vi "RDS Log Reader.vi"() -> ()   [LabVIEW 2015]
uses:
  Actors/RDS Logger Actor/RDS Logger Actor/RDS Logger Actor/Logger Header.ctl
  RDS State Tracker/RDS State/RDS State.lvclass
  Libraries/RDS Child Messages/Mission Messages/Mission Controller State Control.ctl
  RDS Mission Controller Actor/Mission Controller Navigation State.ctl
  RDS Mission Controller Actor/MissionOp.ctl
  RDS State Tracker/RDS State/RDS State.lvclass/RDS State.ctl
  <vilib>/Waveform/WDTFileIO.llb/Export Waveforms To Spreadsheet File (1D).vi
  Log/Log Waveform Processors.lvlib
  RDS Mission Controller Actor/RDS Mission Controller Actor.lvlib
  Libraries/RDS Child Messages/Mission Messages/Mission Controller State Message.lvclass
panel:
  out "Open Log Path":path caption="selected path"
  out "log folder":path caption="selected path"
  in  "Browse Files":bool
  in  "Tree":string(tree)
  in  "Open":bool
  in  "Tab Control":T1(tab)
  out "Battery WF":waveform(dbl)[](graph)
  in  "Batt_Autoscale Y":bool caption="OK Button"
  in  "Nav_Autoscale Y":bool caption="OK Button"
  out "Nav WF":waveform(dbl)[](graph)
  out "Helm":waveform(dbl)[](graph)
  in  "Helm Autoscale Y":bool caption="OK Button"
  out "Speed":waveform(dbl)(graph)
  in  "STBD MCB Autoscale Y":bool caption="OK Button"
  out "STBD WFs":waveform(dbl)[](graph)
  out "Port WFs":waveform(dbl)[](graph)
  in  "Port MCB Autoscale Y":bool caption="OK Button"
  out "Thermal WFs":waveform(dbl)[](graph)
  in  "Thermal Autoscale":bool caption="OK Button"
  out "XY Graph":T2(graph)
  in  "Numeric":i32
  in  "btn_index_mission":bool caption="OK Button"
  out "Mission Controller State":T3 {"Mission"."GPS Longitude" format="%.6g"; "Mission"."GPS Latitude" format="%.6g"}
  out "Mission":refnum<class "RDS State.lvclass">[](array[class])
  out "Header":T6
  in  "stop":bool
  out "size(s)":i32
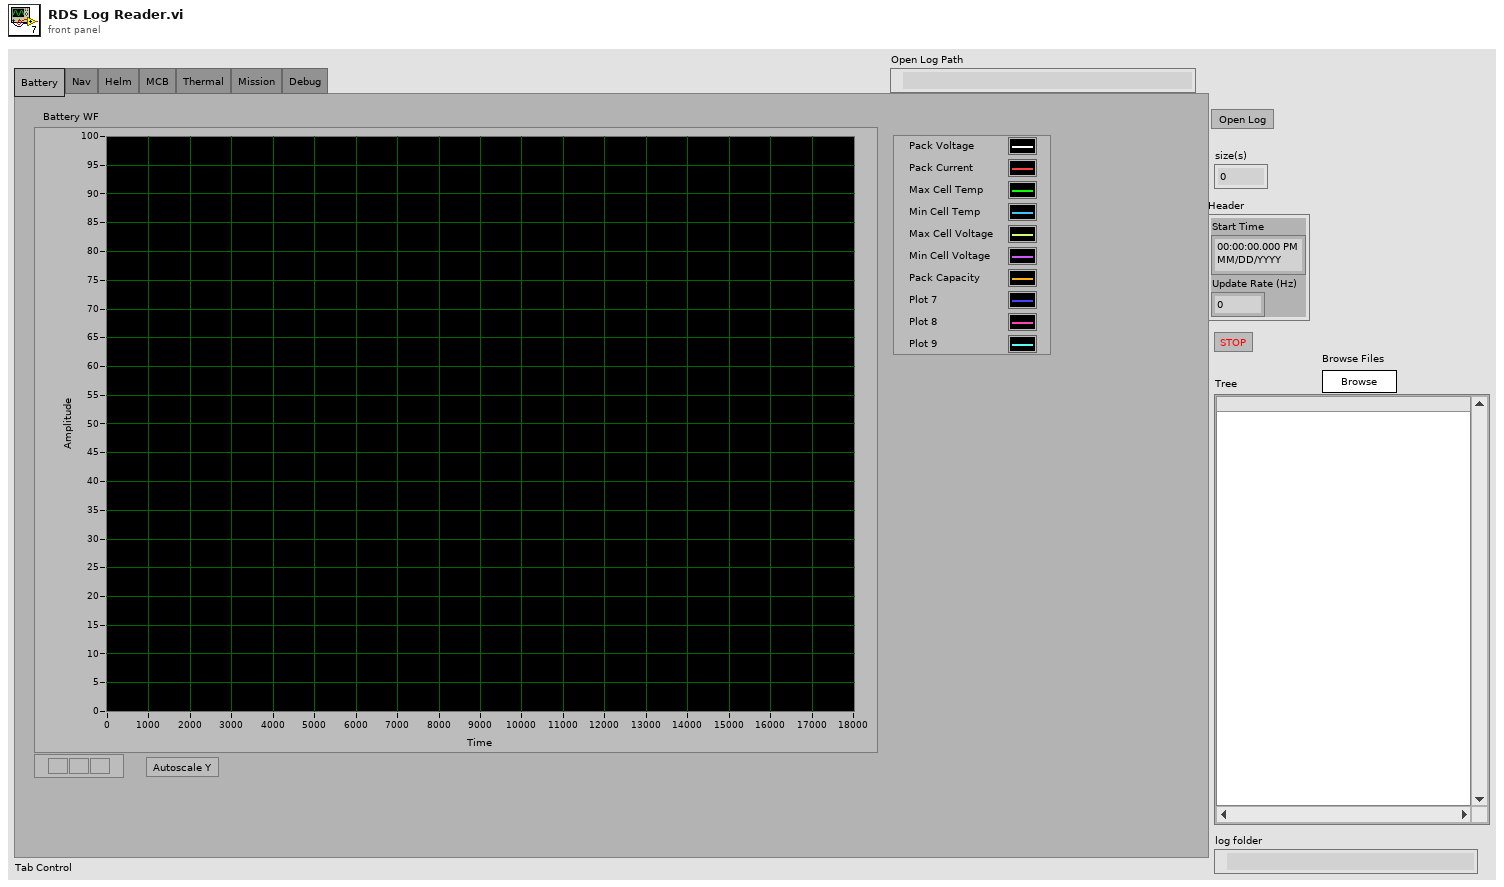
[diagram p1: front panel]
types:
  T1 = enum32{"Battery", "Nav", "Helm", "MCB", "Thermal", "Mission", "Debug"}
  T2 = cluster{"GPS Latitude":ext, "GPS Longitude":ext}[]
  T3 = typedef "RDS Child Messages.lvlib/Mission Controller State Message.lvclass/Mission Controller State Control.ctl" = cluster{"iHasControl":bool, "controlTimer":timestamp, "Nav State":T4, "Current MissionOp Index":i32, "Mission":T5[], "Distance to Target":dbl, "Seconds to Timeout":dbl}
  T4 = typedef "RDS Mission Controller Actor.lvlib/Mission Controller Navigation State.ctl" = cluster{"GPS Latitude":ext, "GPS Longitude":ext, "Compass Heading":dbl, "Speed":dbl}
  T5 = typedef "RDS Mission Controller Actor.lvlib/MissionOp.ctl" = cluster{"MissionOp Type":enum16{"Waypoint", "Loiter", "Wait", "Deploy AIP", "Stow AIP"}, "Duration (s)":u16, "Throttle":i16, "GPS Latitude":dbl, "GPS Longitude":dbl, "Loiter Range (m)":u16}
  T6 = typedef "Log Waveform Processors.lvlib/Logger Header.ctl" = cluster{"Start Time":timestamp, "Update Rate (Hz)":dbl}
  T7 = cluster{"Left Cell String":string, "Child Text":string[], "Child Tag":string, "Item Indent":i32, "Child Only?":bool, "Glyph Index":i32}
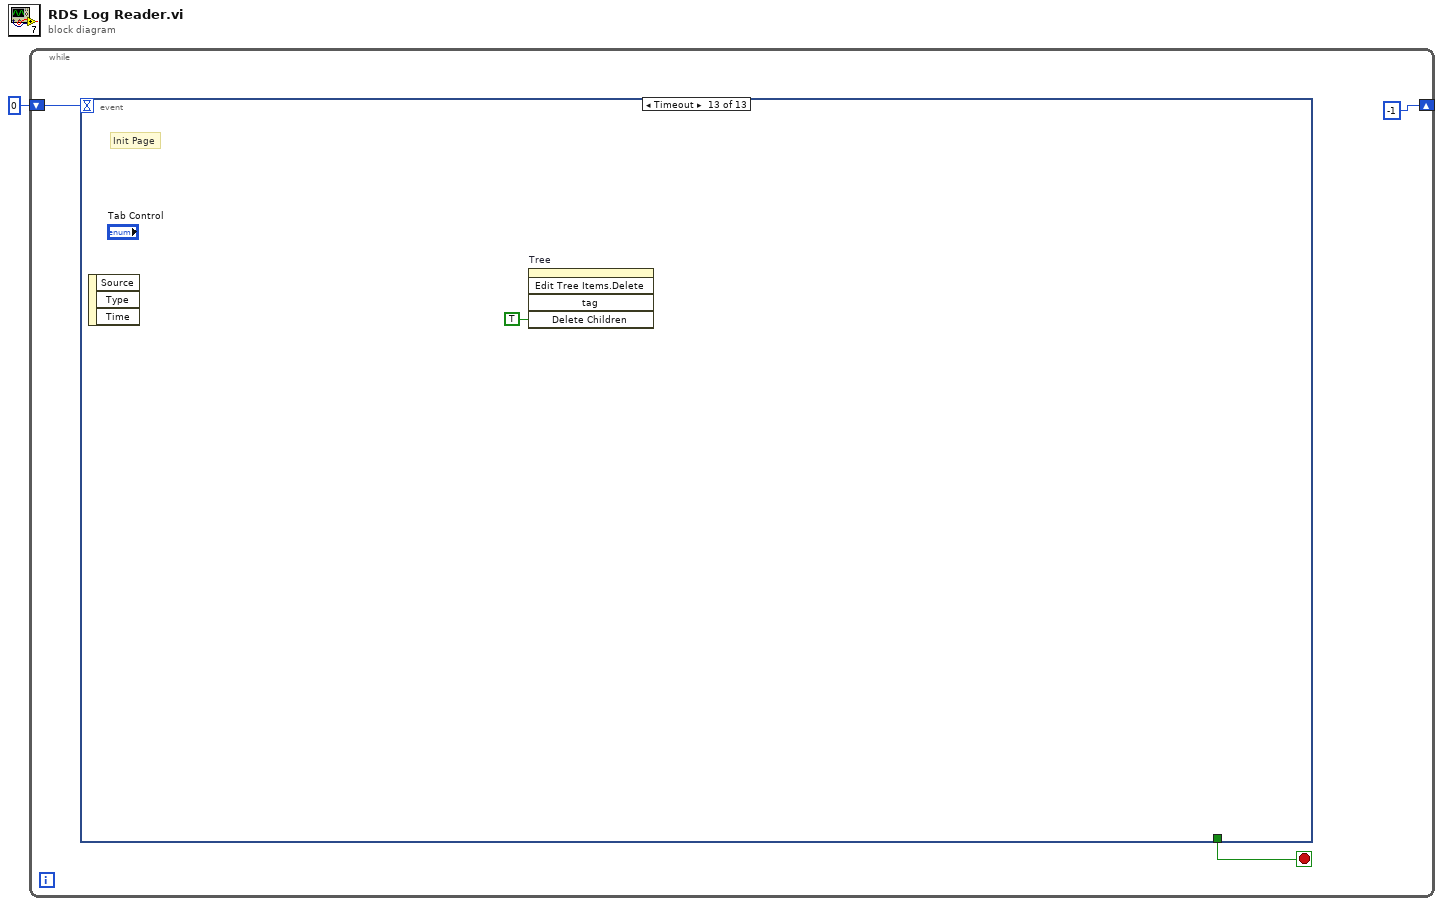
[diagram p0: block diagram]
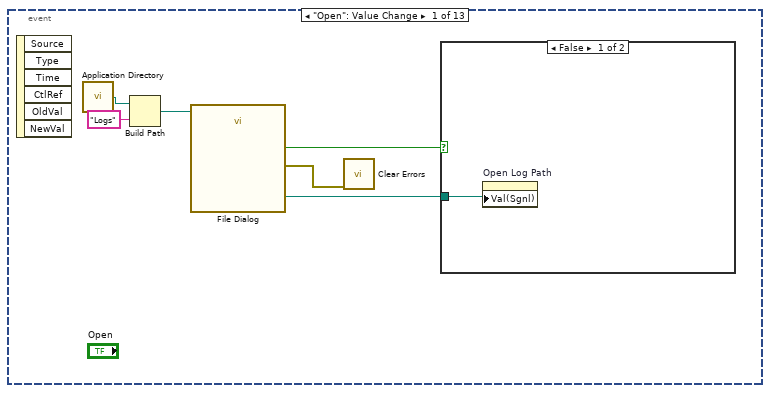
[diagram p2: hidden frame]
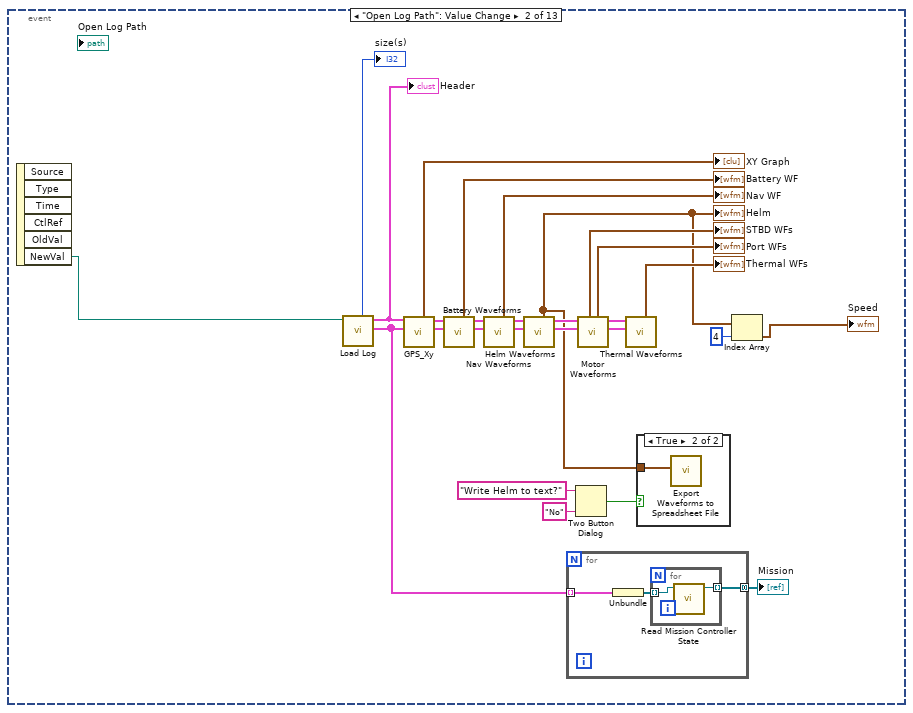
[diagram p4: hidden frame]
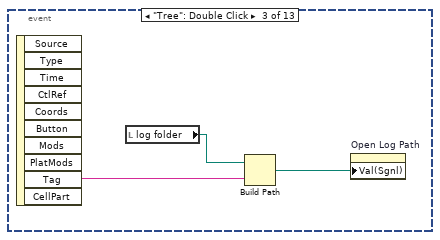
[diagram p6: hidden frame]
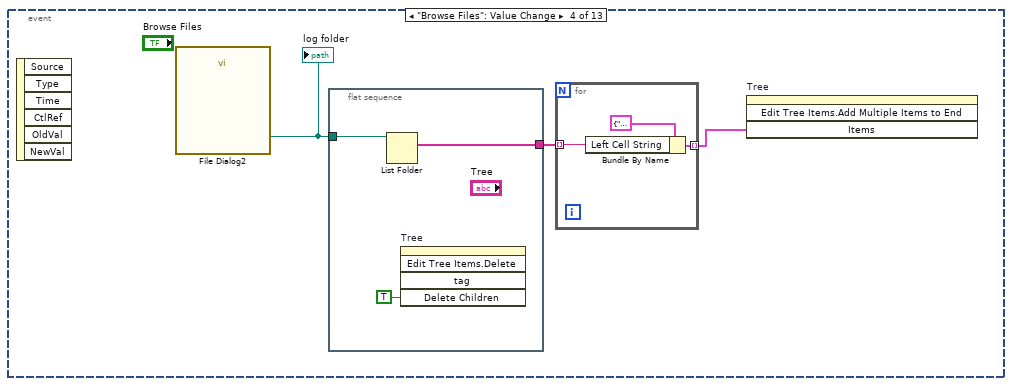
[diagram p7: hidden frame]
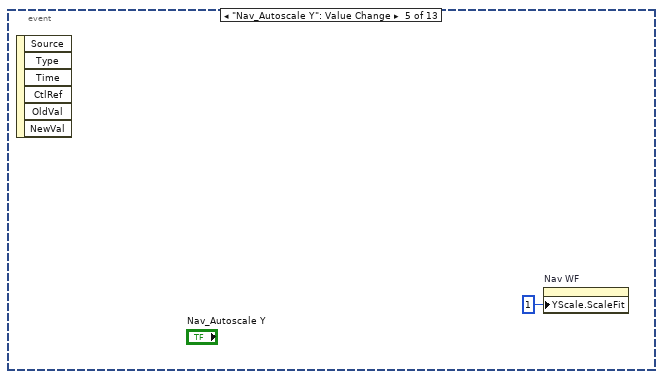
[diagram p8: hidden frame]
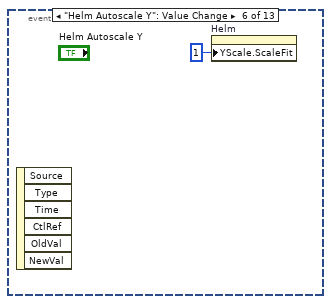
[diagram p9: hidden frame]
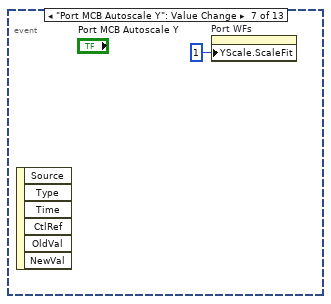
[diagram p10: hidden frame]
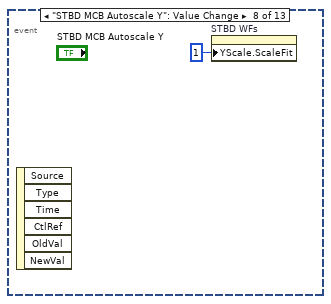
[diagram p11: hidden frame]
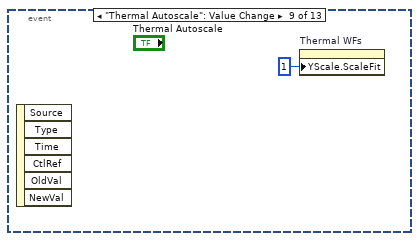
[diagram p12: hidden frame]
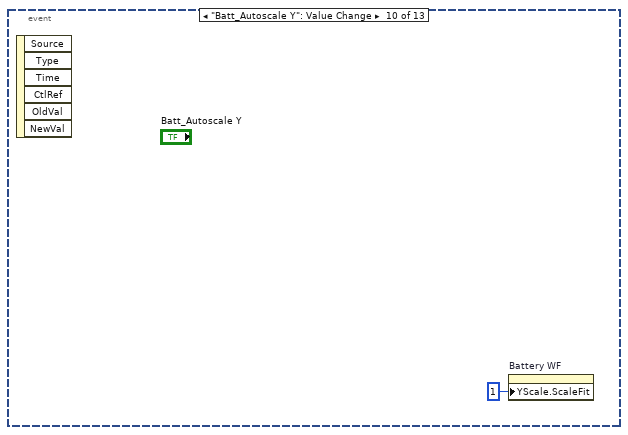
[diagram p13: hidden frame]
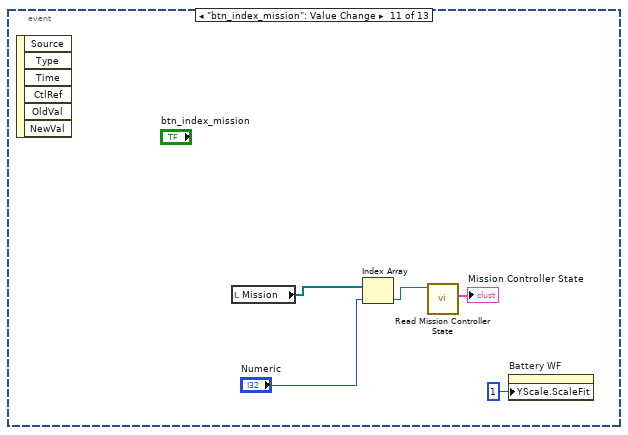
[diagram p14: hidden frame]
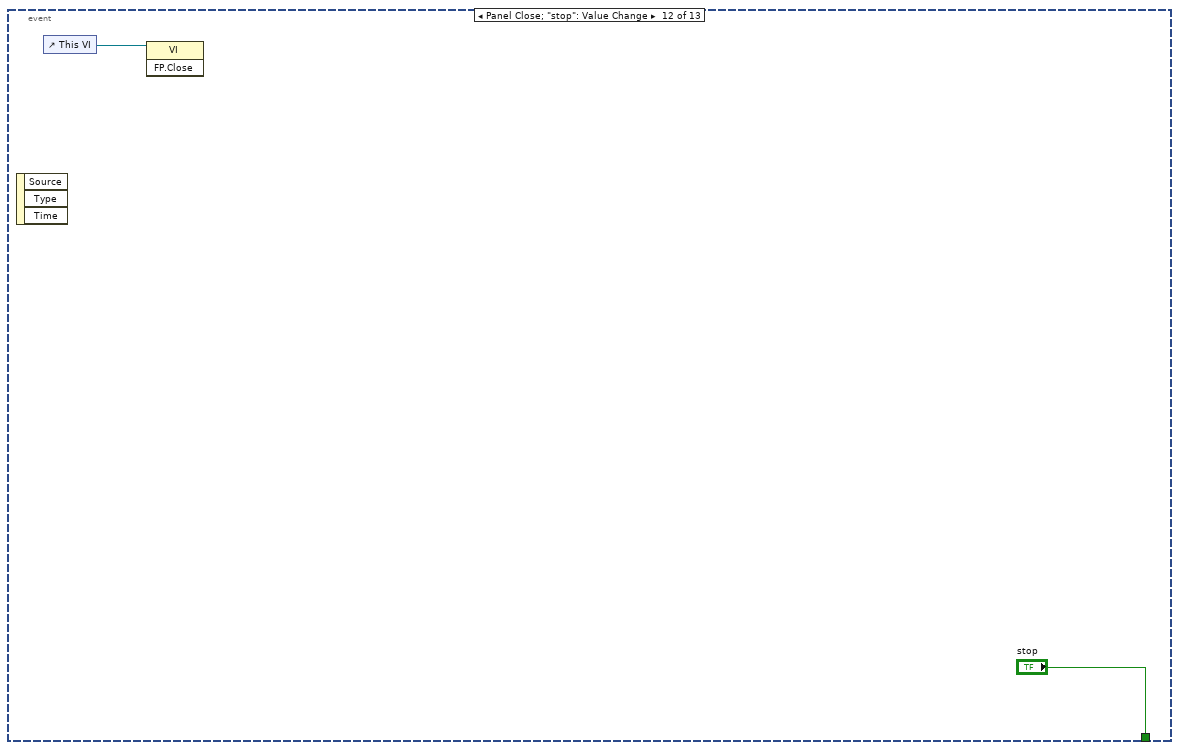
[diagram p15: hidden frame]
diagram:
  n1 = while {
    shift-right: [-1] -> _
    shift-left: 0 -> [w2]
    stop <- w4 stop-if-true
    n2 = event shown="[12] Timeout" {
      selector: _ -> [_ _ _ _ _ _ _ _ _ _ _ _ _]
      dyn-events: _ -> [_ _ _ _ _ _ _ _ _ _ _ _ _]
      timeout: w2 -> [_ _ _ _ _ _ _ _ _ _ _ _ _]
      tunnel: [_ _ _ _ _ _ _ _ _ _ _ "stop" _] -> w4
      event "Open": Value Change {
        n3 = event-data() -> ()  [unwired: 1 in, 6 out]
        n4 = call <vilib>:"Application Directory.vi"() -> ("Application Directory"=w9:path)
        n5 = Build Path(base path=w9, name or relative path="Logs") -> (appended path=w7:path)
        n6 = call "File Dialog"("start path"=w7) -> ("selected path"=w10:path, "cancelled"=w6:bool, "error out"=w5:errorcluster)  [unwired: 11 in, 1 out]
        n7 = call <vilib>:"Clear Errors.vi"("error in (no error)"=w5) -> ()  [unwired: 5 in, 2 out]
        n8 = case shown="False" w6 {
          tunnel: w10 -> [w11 _]
          frame False {
            n9 = property on="Open Log Path" class="Path"("Val(Sgnl)"=w11) -> ()  [unwired: 2 in, 2 out]
          }
          frame True {
          }
        }
      }
      event "Open Log Path": Value Change {
        n10 = event-data() -> ("NewVal"=w15:path)  [unwired: 1 in, 5 out]
        n11 = call "Load Log.vi"("selected path"=w15) -> ("Log Data"=w25:cluster{refnum<class "RDS State.lvclass">[]}[], "Log Header"=w24:T6, "size(s)"=→"size(s)":i32)  [unwired: 8 in]
        "Header" <- w24
        n12 = call "GPS_Xy.vi"("Log Data In"=w25, "Log Header"=w24) -> ("Log Data Out"=w32:cluster{refnum<class "RDS State.lvclass">[]}[], "Log Header Out"=w33:T6, "Lat Long"=→"XY Graph":T2)  [unwired: 7 in]
        n13 = call "Battery Waveforms.vi"("Log Read Data"=w32, "Header"=w33) -> ("Log Data Out"=w28:cluster{refnum<class "RDS State.lvclass">[]}[], "Header Out"=w29:T6, "Battery WFs"=→"Battery WF":waveform(dbl)[])  [unwired: 7 in]
        n14 = call "Nav Waveforms.vi"("Log Data In"=w28, "Log Header"=w29) -> ("Log Data Out"=w26:cluster{refnum<class "RDS State.lvclass">[]}[], "Log Header Out"=w27:T6, "Nav Data Out"=→"Nav WF":waveform(dbl)[])  [unwired: 7 in]
        n15 = call "Helm Waveforms.vi"("Log Data In"=w26, "Log Header In"=w27) -> ("Log Data Out"=w22:cluster{refnum<class "RDS State.lvclass">[]}[], "Log Header Out"=w23:T6, "Heading Command"=w14:waveform(dbl)[])  [unwired: 7 in]
        "Helm" <- w14
        n16 = for {
          tunnel: [w41] -> w38 mode=concatenating
          tunnel: w25 -> [w40] mode=indexing
          n17 = Unbundle(w40) -> (w42:refnum<class "RDS State.lvclass">[])
          n18 = for {
            tunnel: w42 -> [w44] mode=indexing
            tunnel: [w43] -> w41 mode=indexing
            n19 = call "Read Mission Controller State.vi"("RDS State in"=w44) -> ("RDS State out"=w43:refnum<class "RDS State.lvclass">)  [unwired: 8 in, 2 out]
          }
        }
        "Mission" <- w38
        n20 = Two Button Dialog(message="Write Helm to text?", 1:"No" ("F button name (\"Cancel\")")) -> (T button?=w37:bool)  [unwired: 1 in]
        n21 = call "Motor Waveforms.vi"("Log Data in"=w22, "Log Header In"=w23) -> ("Log Data out"=w19:cluster{refnum<class "RDS State.lvclass">[]}[], "Log Header Out"=w18:T6, "STBD Motor WFs"=→"Port WFs":waveform(dbl)[], "Port Motor WFs"=→"STBD WFs":waveform(dbl)[])  [unwired: 6 in]
        n22 = call "Thermal Waveforms.vi"("Log Read Data"=w19, "Header"=w18) -> ("Thermal WFs"=→"Thermal WFs":waveform(dbl)[])  [unwired: 7 in, 2 out]
        n23 = case shown="True" w37 {
          tunnel: w14 -> [_ w39]
          frame False {
          }
          frame True {
            n24 = call-poly <vilib>:"Export Waveforms to Spreadsheet File.vi"("waveforms"=w39) -> ()  [unwired: 9 in, 2 out]
          }
        }
        n25 = Index Array(array=w14, index=4) -> (element=→"Speed":waveform(dbl))
      }
      event "Tree": Double Click {
        n26 = event-data() -> ("Tag"=w47:string)  [unwired: 1 in, 9 out]
        n27 = local read "log folder"() -> (w46:path)
        n28 = Build Path(base path=w46, name or relative path=w47) -> (appended path=w45:path)
        n29 = property on="Open Log Path" class="Path"("Val(Sgnl)"=w45) -> ()  [unwired: 2 in, 2 out]
      }
      event "Browse Files": Value Change {
        n30 = event-data() -> ()  [unwired: 1 in, 6 out]
        n31 = call "File Dialog2"() -> ("selected path"=w49:path)  [unwired: 12 in, 3 out]
        "log folder" <- w49
        n32 = flat-sequence {
          tunnel: [w53] -> w50
          tunnel: w49 -> [w52]
          frame #0 {
            n33 = List Folder(path=w52) -> (filenames=w53:string[])  [unwired: 3 in, 3 out]
            n34 = invoke on="Tree" class="Tree (strict)" method="Edit Tree Items.Delete"("Delete Children"=TRUE ("Delete Children?")) -> ()  [unwired: 4 in, 5 out]
          }
        }
        n35 = for {
          tunnel: w50 -> [w56] mode=indexing
          tunnel: [w55] -> w48 mode=indexing
          n36 = Bundle By Name(cluster=T7 {"Left Cell String"="", "Child Text"=[], "Child Tag"="", "Item Indent"=0, "Child Only?"=FALSE, "Glyph Index"=0} ("Item"), "Left Cell String"=w56) -> (w55:T7)
        }
        n37 = invoke on="Tree" class="Tree (strict)" method="Edit Tree Items.Add Multiple Items to End"("Items"=w48) -> ()  [unwired: 3 in, 4 out]
      }
      event "Nav_Autoscale Y": Value Change {
        n38 = event-data() -> ()  [unwired: 1 in, 6 out]
        n39 = property on="Nav WF" class="WFGraph (strict)"("YScale.ScaleFit"=u8 1 ("X Scale.Scale Fit")) -> ()  [unwired: 2 in, 2 out]
      }
      event "Helm Autoscale Y": Value Change {
        n40 = event-data() -> ()  [unwired: 1 in, 6 out]
        n41 = property on="Helm" class="WFGraph (strict)"("YScale.ScaleFit"=u8 1 ("X Scale.Scale Fit")) -> ()  [unwired: 2 in, 2 out]
      }
      event "Port MCB Autoscale Y": Value Change {
        n42 = event-data() -> ()  [unwired: 1 in, 6 out]
        n43 = property on="Port WFs" class="WFGraph (strict)"("YScale.ScaleFit"=u8 1 ("X Scale.Scale Fit")) -> ()  [unwired: 2 in, 2 out]
      }
      event "STBD MCB Autoscale Y": Value Change {
        n44 = event-data() -> ()  [unwired: 1 in, 6 out]
        n45 = property on="STBD WFs" class="WFGraph (strict)"("YScale.ScaleFit"=u8 1 ("X Scale.Scale Fit")) -> ()  [unwired: 2 in, 2 out]
      }
      event "Thermal Autoscale": Value Change {
        n46 = event-data() -> ()  [unwired: 1 in, 6 out]
        n47 = property on="Thermal WFs" class="WFGraph (strict)"("YScale.ScaleFit"=u8 1 ("X Scale.Scale Fit")) -> ()  [unwired: 2 in, 2 out]
      }
      event "Batt_Autoscale Y": Value Change {
        n48 = event-data() -> ()  [unwired: 1 in, 6 out]
        n49 = property on="Battery WF" class="WFGraph (strict)"("YScale.ScaleFit"=u8 1 ("X Scale.Scale Fit")) -> ()  [unwired: 2 in, 2 out]
      }
      event "btn_index_mission": Value Change {
        n50 = event-data() -> ()  [unwired: 1 in, 6 out]
        n51 = local read "Mission"() -> (w65:refnum<class "RDS State.lvclass">[])
        n52 = Index Array(array=w65, index="Numeric") -> (element=w64:refnum<class "RDS State.lvclass">)
        n53 = call "Read Mission Controller State.vi"("RDS State in"=w64) -> ("Mission Controller State"=→"Mission Controller State":T3)  [unwired: 8 in, 2 out]
        n54 = property on="Battery WF" class="WFGraph (strict)"("YScale.ScaleFit"=u8 1 ("X Scale.Scale Fit")) -> ()  [unwired: 2 in, 2 out]
      }
      event Panel Close; "stop": Value Change {
        n55 = event-data() -> ()  [unwired: 1 in, 3 out]
        n56 = control-ref of="This VI"() -> (w68:refnum<vi>)
        n57 = invoke class="VI" method="FP.Close"(reference=w68) -> ()  [unwired: 2 in, 3 out]
      }
      event Timeout {
        # "Init Page"
        n58 = event-data() -> ()  [unwired: 1 in, 3 out]
        n59 = invoke on="Tree" class="Tree (strict)" method="Edit Tree Items.Delete"("Delete Children"=TRUE ("Delete Children?")) -> ()  [unwired: 4 in, 5 out]
      }
    }
  }
